vi "Configure CPC.vi"(8 "error in":errorcluster, 10 "Config Handle":T1) -> (0 "error out":errorcluster, 3 "CPC out":refnum<class "CPC.lvclass">)   [LabVIEW 2014, in "CPC.lvclass"]
uses:
  CPC.lvclass
  reusable/Session APIs/Serial/Serial Session.lvclass
  reusable/Session APIs/File Access/Config Data/Config Data.lvclass
  <vilib>/Utility/config.llb/NI_LVConfig.lvlib
  <vilib>/Utility/config.llb/Read Key (String).vi
  <vilib>/Utility/config.llb/Read Key (Boolean).vi
  reusable/Session APIs/File Access/Config Data/Config Session.ctl
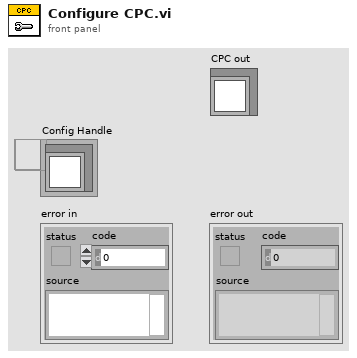
[diagram p1: front panel]
types:
  T1 = typedef "Config Data.lvclass/Config Session.ctl" = refnum<data-value>
  T2 = typedef "Serial Session.lvclass/Session Handle.ctl" = refnum<data-value>
  T3 = typedef "NI_LVConfig.lvlib/Config Data RefNum.ctl" = refnum<k1>
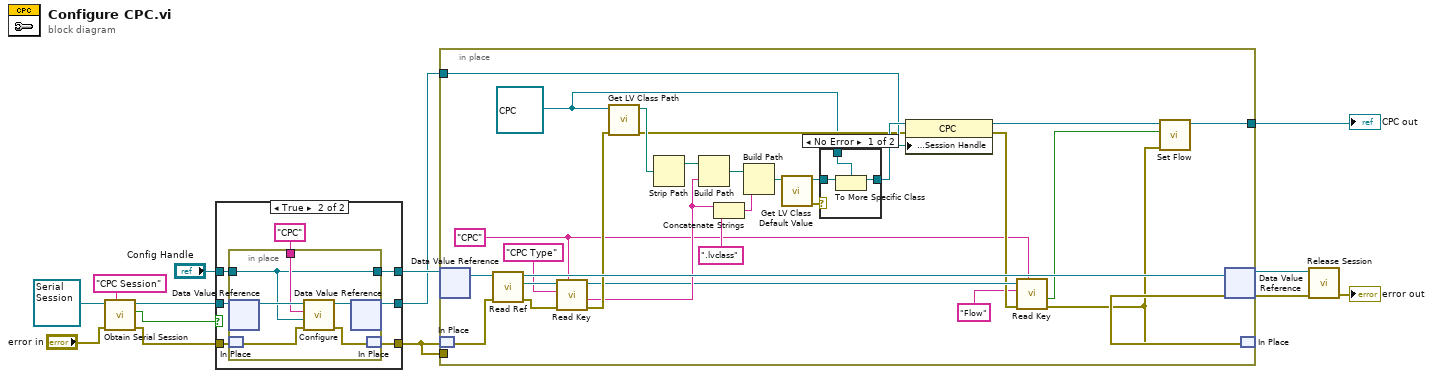
[diagram p0: block diagram]
diagram:
  n1 = call "Obtain Serial Session.vi"("Session Name ()"="CPC Session", "error in"="error in", "Serial Session in"=refnum<class "Serial Session.lvclass"> refnum) -> ("error out"=w8:errorcluster, "created new?"=w3:bool, "hSerial"=w13:T2)  [unwired: 6 in]
  n2 = case shown="True" w3 {
    tunnel: w13 -> [w17 w24]
    tunnel: w8 -> [w16 w20]
    tunnel: [w17 w23] -> w7
    tunnel: [w16 w22] -> w1
    tunnel: "Config Handle" -> [w15 w21]
    tunnel: [w15 w19] -> w11
    frame False {
    }
    frame True {
      n3 = in-place {
        in-place-border: w21 -> [w25]
        in-place-border: "CPC" ("section") -> [w26]
        in-place-border: [w25] -> w19
        n4 = in-place-dvr #1(w24) -> (w30:refnum<class "Serial Session.lvclass">)  [unwired: 1 out]
        n5 = in-place-match #2(w20) -> (w29:errorcluster)
        n6 = call "Configure.vi"("error in"=w29, "Config Handle"=w25, "section"=w26, "Serial Session in"=w30) -> ("error out"=w28:errorcluster, "Serial Session out"=w27:refnum<class "Serial Session.lvclass">)  [unwired: 6 in]
        n7 = in-place-dvr #1(w27) -> (w23:T2)  [unwired: 1 out]
        n8 = in-place-match #2(w28) -> (w22:errorcluster)
      }
    }
  }
  n9 = in-place {
    in-place-border: w7 -> [w42]
    in-place-border: [w33] -> w4
    in-place-border: w1 -> [_]
    w36 = refnum<class "CPC.lvclass"> refnum ("CPC in")
    w38 = "CPC" ("section")
    n10 = in-place-dvr #3(w11) -> (w58:refnum<class "Config Data.lvclass">)  [unwired: 1 out]
    n11 = in-place-match #4(w1) -> (w35:errorcluster)
    n12 = call "Read Ref.vi"("error in"=w35, "Config Data in"=w58) -> ("error out"=w56:errorcluster, "config data"=w57:T3, "Config Data out"=w55:refnum<class "Config Data.lvclass">)  [unwired: 7 in]
    n13 = call-poly <vilib>:"Read Key.vi"("section"=w38, "error in (no error)"=w56, "key"="CPC Type", "refnum"=w57) -> ("error out"=w53:errorcluster, "value"=w49:string, "refnum out"=w40:T3)  [unwired: 4 in, 1 out]
    n14 = call <vilib>:"Get LV Class Path.vi"("error in (no error)"=w53, "object"=w36) -> ("error out"=w41:errorcluster, "class path"=w52:path)  [unwired: 8 in]
    n15 = Strip Path(path=w52) -> (stripped path=w51:path)  [unwired: 1 out]
    n16 = Build Path(base path=w51, name or relative path=w49) -> (appended path=w50:path)
    n17 = Concatenate Strings(w49, ".lvclass" ("string")) -> (w47:string)
    n18 = Build Path(base path=w50, name or relative path=w47) -> (appended path=w46:path)
    n19 = call <vilib>:"Get LV Class Default Value.vi"("class path"=w46) -> ("error out"=w44:errorcluster, "object"=w45:refnum<class>)  [unwired: 9 in]
    n20 = case shown="No Error" w44 {
      tunnel: w45 -> [w61 _]
      tunnel: [w60 w62] -> w43
      tunnel: w36 -> [w59 w62]
      frame No Error {
        n21 = To More Specific Class(target class=w59, reference=w61) -> (specific class reference=w60:refnum<class "CPC.lvclass">)  [unwired: 1 in, 1 out]
      }
      frame Error {
      }
    }
    n22 = property class="CPC"(reference=w43, error in=w41, "Accessors:Session Handle"=w42) -> (reference out=w34:refnum<class "CPC.lvclass">, error out=w39:errorcluster)
    n23 = call-poly <vilib>:"Read Key.vi"("section"=w38, "error in (no error)"=w39, "key"="Flow", "refnum"=w40) -> ("error out"=w31:errorcluster, "value"=w32:bool)  [unwired: 4 in, 2 out]
    n24 = call-dynamic "Set Flow.vi"("error in"=w31, "High Flow?"=w32, "CPC in"=w34) -> ("CPC out"=w33:refnum<class "CPC.lvclass">)  [unwired: 7 in, 1 out]
    n25 = in-place-dvr #3(w55) -> (w6:T1)  [unwired: 1 out]
    n26 = in-place-match #4(w31) -> (w5:errorcluster)
  }
  "CPC out" <- w4
  n27 = call "Release Session.vi"("error in"=w5, "Session Handle"=w6) -> ("error out"=→"error out":errorcluster)  [unwired: 8 in, 1 out]
